vi "CRYSet ViewProperty Misc Front Panel.vi"(11 "Vi Ref":refnum<vi>) -> ()   [LabVIEW 2013]
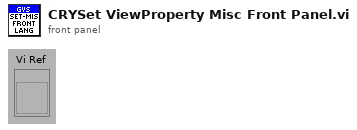
[diagram p1: front panel]
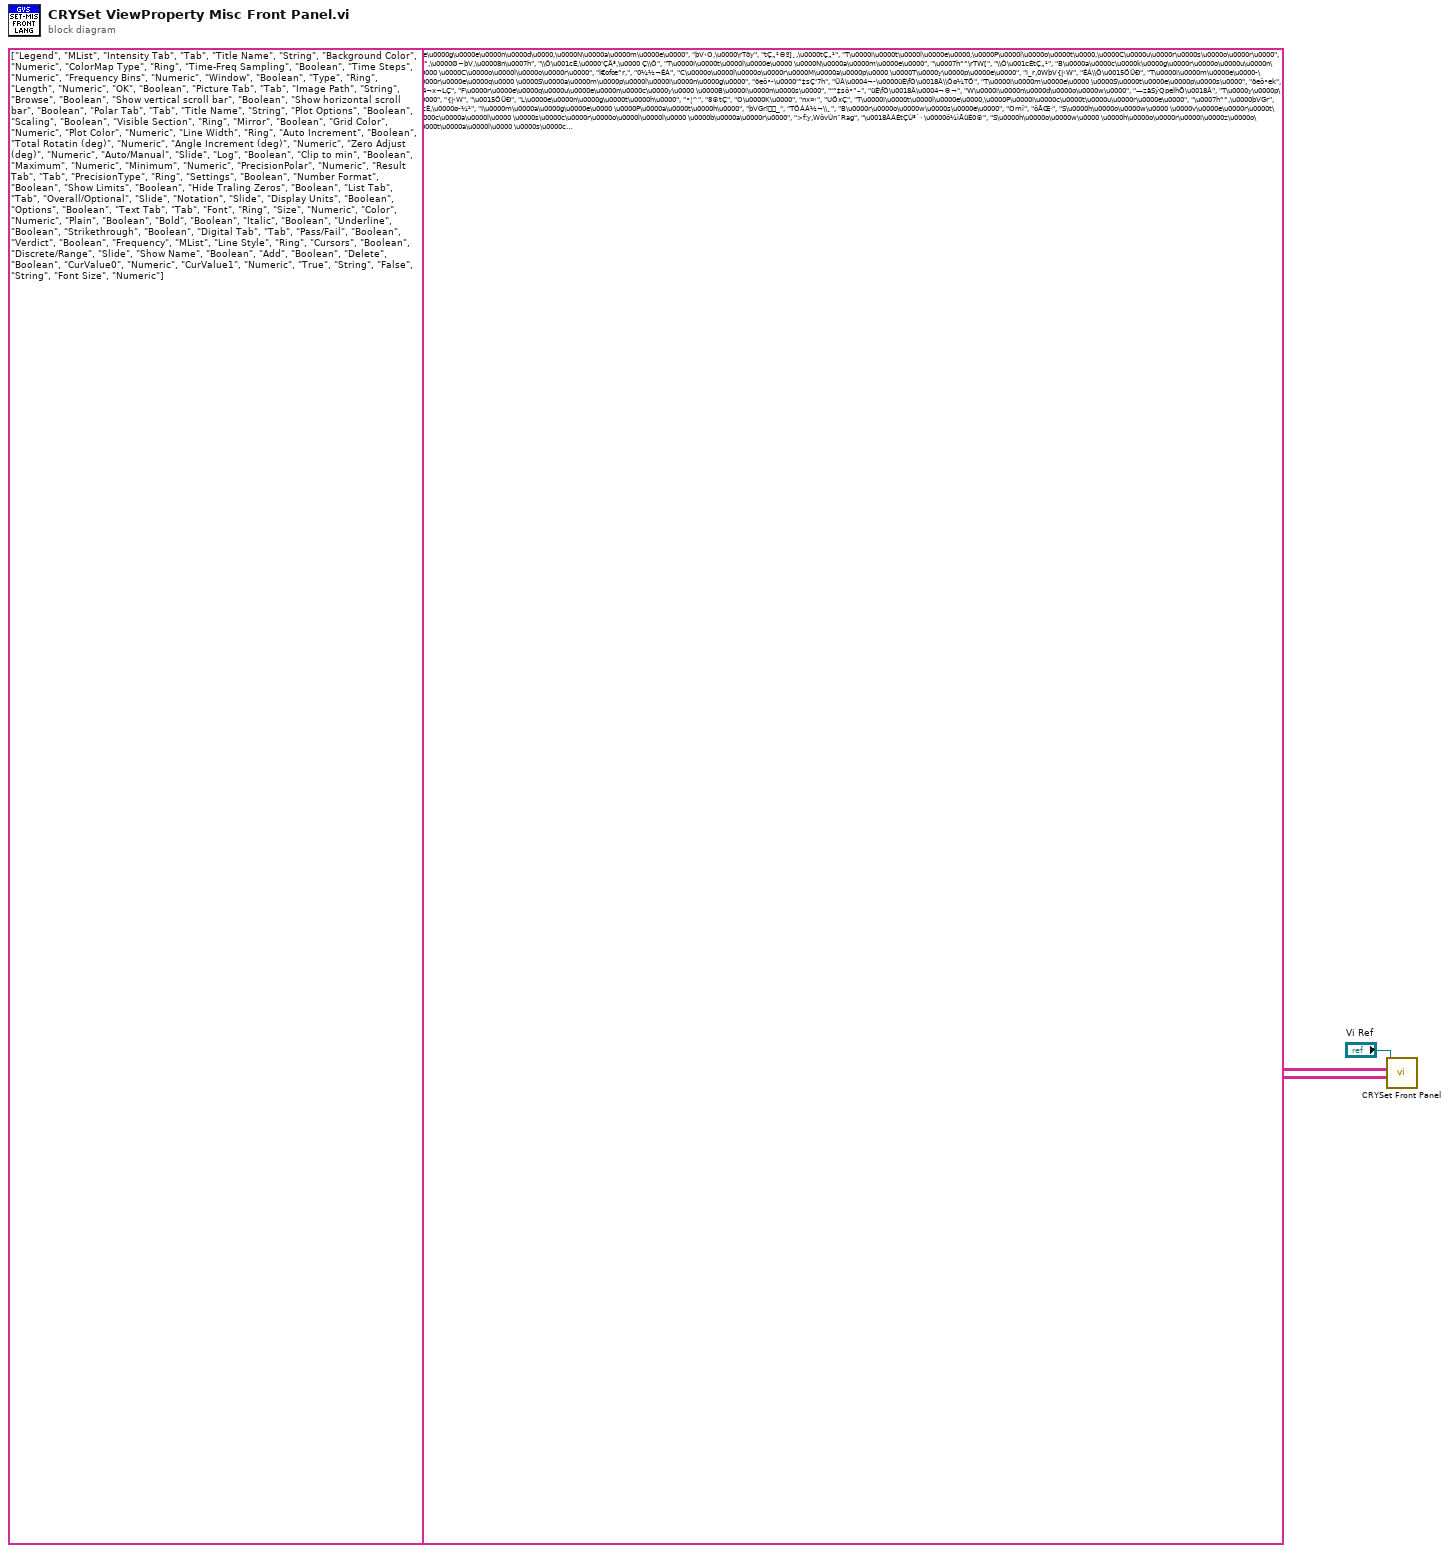
[diagram p0: block diagram]
diagram:
  # "Caption, Tab Page, Multilist Header, Button 4"
  # "Control Type"
  # "Control Name and Tab"
  # "caption, boolean text(,,,)"
  # "Caption/Boolean Text"
  n1 = call "CRYSet Front Panel.vi"("Caption(Boolean Text)"=string[][] [["L\u0000e\u0000g\u0000e\u0000n\u0000d\u0000,\u0000N\u0000a\u0000m\u0000e\u0000", "þV‹O,\u0000\rTðy", "tÇ„¹©º]¸,\u0000tÇ„¹"], ["T\u0000i\u0000t\u0000l\u0000e\u0000,\u0000P\u0000l\u0000o\u0000t\u0000,\u0000C\u0000u\u0000r\u0000s\u0000o\u0000r\u0000", "\u0007h˜˜,\u0000Ø~þV,\u00008n\u0007h", "\\Ô\u001cÈ,\u0000‘ÇÄ³,\u0000 Ç\\Ô"], ["T\u0000i\u0000t\u0000l\u0000e\u0000 \u0000N\u0000a\u0000m\u0000e\u0000", "\u0007h˜˜\rTW[", "\\Ô\u001cÈtÇ„¹"], ["B\u0000a\u0000c\u0000k\u0000g\u0000r\u0000o\u0000u\u0000n\u0000d\u0000 \u0000C\u0000o\u0000l\u0000o\u0000r\u0000", "Ì€ofœ˜r‚", "0¼½¬ÉÀ"], ["C\u0000o\u0000l\u0000o\u0000r\u0000M\u0000a\u0000p\u0000 \u0000T\u0000y\u0000p\u0000e\u0000", "i_r‚0WþV{|‹W", "ÉÀ\\Ô\u0015ÖÜÐ"], ["T\u0000i\u0000m\u0000e\u0000-\u0000F\u0000r\u0000e\u0000q\u0000 \u0000S\u0000a\u0000m\u0000p\u0000l\u0000i\u0000n\u0000g\u0000", "öeô•-\u0000‘˜‡sÇ‘7h", "ÜÂ\u0004¬-\u0000üÈ\fÓ\u0018Â\\Ôø¼TÖ"], ["T\u0000i\u0000m\u0000e\u0000 \u0000S\u0000t\u0000e\u0000p\u0000s\u0000", "öeô•ek", "ÜÂ\u0004¬x¬LÇ"], ["F\u0000r\u0000e\u0000q\u0000u\u0000e\u0000n\u0000c\u0000y\u0000 \u0000B\u0000i\u0000n\u0000s\u0000", "‘˜‡sô•”–", "üÈ\fÓ\u0018Â\u0004¬©¬"], ["W\u0000i\u0000n\u0000d\u0000o\u0000w\u0000", "—zãSýQpe", "=ÌhÕ\u0018Â"], ["T\u0000y\u0000p\u0000e\u0000", "{|‹W", "\u0015ÖÜÐ"], ["L\u0000e\u0000n\u0000g\u0000t\u0000h\u0000", "•¦^", "8®tÇ"], ["O\u0000K\u0000", "nx¤‹", "UÖxÇ"], ["T\u0000i\u0000t\u0000l\u0000e\u0000,\u0000P\u0000i\u0000c\u0000t\u0000u\u0000r\u0000e\u0000", "\u0007h˜˜,\u0000þVGr", "\\Ô\u001cÈ,\u0000ø­¼¹"], ["I\u0000m\u0000a\u0000g\u0000e\u0000 \u0000P\u0000a\u0000t\u0000h\u0000", "þVGrï_", "TÖÁÀ½¬\\¸"], ["B\u0000r\u0000o\u0000w\u0000s\u0000e\u0000", "Omȉ", "ôÅŒ·"], ["S\u0000h\u0000o\u0000w\u0000 \u0000v\u0000e\u0000r\u0000t\u0000i\u0000c\u0000a\u0000l\u0000 \u0000s\u0000c\u0000r\u0000o\u0000l\u0000l\u0000 \u0000b\u0000a\u0000r\u0000", ">f:y‚WôvÚn¨Rag", "\u0018ÂÁÉtÇÙ³`· \u0000ô¼ìÅüÈ0®"], ["S\u0000h\u0000o\u0000w\u0000 \u0000h\u0000o\u0000r\u0000i\u0000z\u0000o\u0000n\u0000t\u0000a\u0000l\u0000 \u0000s\u0000c\u0000r\u0000o\u0000l\u0000l\u0000 \u0000b\u0000a\u0000r\u0000", ">f:y4ls^Ún¨Rag", "\u0018ÂÉÓtÇÙ³`· \u0000ô¼ìÅüÈ0®"], ["T\u0000i\u0000t\u0000l\u0000e\u0000,\u0000P\u0000l\u0000o\u0000t\u0000,\u0000X\u0000Y\u0000 \u0000G\u0000r\u0000a\u0000p\u0000h\u0000", "\u0007h˜˜,\u0000Ø~þV,\u0000X\u0000Y\u0000þVhˆ", "\\Ô\u001cÈ,\u0000‘ÇÄ³,\u0000X\u0000Y\u0000ø­|·\u0004Õ"], ["T\u0000i\u0000t\u0000l\u0000e\u0000 \u0000N\u0000a\u0000m\u0000e\u0000", "\u0007h˜˜\rTW[", "\\Ô\u001cÈtÇ„¹"], ["P\u0000l\u0000o\u0000t\u0000 \u0000O\u0000p\u0000t\u0000i\u0000o\u0000n\u0000s\u0000", "Ø~þV\ty", "‘ÇÄ³ ÁÝÐmÕ©º"], ["S\u0000c\u0000a\u0000l\u0000i\u0000n\u0000g\u0000", ")>e", "™ÌÄ³"], ["V\u0000i\u0000s\u0000i\u0000b\u0000l\u0000e\u0000 \u0000S\u0000e\u0000c\u0000t\u0000i\u0000o\u0000n\u0000", "ïSÁè\u0006R", "ô¼„Çl­íÅ"], ["M\u0000i\u0000r\u0000r\u0000o\u0000r\u0000", "\\•P[ÍS\u0004\\", "p¬¸Æ\u0018¼¬À"], ["G\u0000r\u0000i\u0000d\u0000 \u0000C\u0000o\u0000l\u0000o\u0000r\u0000", "Q<hœ˜r‚", "©¬ÇÉÀ\b¬"], ["P\u0000l\u0000o\u0000t\u0000 \u0000C\u0000o\u0000l\u0000o\u0000r\u0000", "Ø~þVœ˜r‚", " Á \u0000ÉÀ\b¬"], ["L\u0000i\u0000n\u0000e\u0000 \u0000W\u0000i\u0000d\u0000t\u0000h\u0000", "Ø~þV¿~½[¦^", " Á \u0000\b±D¾"], ["A\u0000u\u0000t\u0000o\u0000 \u0000I\u0000n\u0000c\u0000r\u0000e\u0000m\u0000e\u0000n\u0000t\u0000", "ê¨RXÏ", "ÇÙ³É\u0000¬"], ["T\u0000o\u0000t\u0000a\u0000l\u0000 \u0000R\u0000o\u0000t\u0000a\u0000t\u0000i\u0000n\u0000 \u0000(\u0000d\u0000e\u0000g\u0000)\u0000", "hQSOÞVl(\u0000¦^)\u0000", "\u0004È´ÌŒÖ\u0004È(\u0000Ä³)\u0000"], ["A\u0000n\u0000g\u0000l\u0000e\u0000 \u0000I\u0000n\u0000c\u0000r\u0000e\u0000m\u0000e\u0000n\u0000t\u0000 \u0000(\u0000d\u0000e\u0000g\u0000)\u0000", "Ò‰¦^žXÏ‘(\u0000¦^)\u0000", "\u0001¬É½(\u0000Ä³)\u0000"], ["Z\u0000e\u0000r\u0000o\u0000 \u0000A\u0000d\u0000j\u0000u\u0000s\u0000t\u0000 \u0000(\u0000d\u0000e\u0000g\u0000)\u0000", "\u0003Œö–(\u0000¦^)\u0000", "9¸pÈ\bÈ(\u0000Ä³)\u0000"], ["A\u0000u\u0000t\u0000o\u0000/\u0000M\u0000a\u0000n\u0000u\u0000a\u0000l\u0000,\u0000A\u0000u\u0000t\u0000o\u0000,\u0000M\u0000a\u0000n\u0000u\u0000a\u0000l\u0000", "A\u0000u\u0000t\u0000o\u0000/\u0000M\u0000a\u0000n\u0000u\u0000a\u0000l\u0000,\u0000ê¨R,\u0000Kb¨R", "ÇÙ³/\u0000\u0018ÂÙ³,\u0000ÇÙ³,\u0000\u0018ÂÙ³"], ["L\u0000o\u0000g\u0000", "ù[pe", "\\¸ø­"], ["C\u0000l\u0000i\u0000p\u0000 \u0000t\u0000o\u0000 \u0000m\u0000i\u0000n\u0000", "jR\u0000gNO", "\\ÍÁÇ¹"], ["M\u0000a\u0000x\u0000i\u0000m\u0000u\u0000m\u0000", "\u0000g'Y<P", "\\Í\u0000³\u0012¬"], ["M\u0000i\u0000n\u0000i\u0000m\u0000u\u0000m\u0000", "\u0000g\u000f\\<P", "\\ÍŒÁ\u0012¬"], ["P\u0000r\u0000e\u0000c\u0000i\u0000s\u0000i\u0000o\u0000n\u0000", "¾|¦^", "\u0015È\u0000¼Ä³"], ["T\u0000i\u0000t\u0000l\u0000e\u0000,\u0000F\u0000o\u0000r\u0000m\u0000a\u0000t\u0000", "\u0007h˜˜,\u0000<h\u000f_", "\\Ô\u001cÈ,\u0000\u0015ÖÝÂ"], ["P\u0000r\u0000e\u0000c\u0000i\u0000s\u0000i\u0000o\u0000n\u0000T\u0000y\u0000p\u0000e\u0000,\u0000D\u0000i\u0000g\u0000i\u0000t\u0000a\u0000l\u0000s\u0000 \u0000o\u0000f\u0000 \u0000p\u0000r\u0000e\u0000c\u0000i\u0000s\u0000i\u0000o\u0000n\u0000,\u0000S\u0000i\u0000g\u0000n\u0000i\u0000f\u0000i\u0000c\u0000a\u0000n\u0000t\u0000 \u0000d\u0000i\u0000g\u0000i\u0000t\u0000s\u0000 \u0000", "¾|¦^,\u0000¾|¦^MOpe,\u0000\tgHepeW[", "\u0015È\u0000¼Ä³,\u0000D\u0000i\u0000g\u0000i\u0000t\u0000a\u0000l\u0000s\u0000 \u0000o\u0000f\u0000 \u0000p\u0000r\u0000e\u0000c\u0000i\u0000s\u0000i\u0000o\u0000n\u0000,\u0000S\u0000i\u0000g\u0000n\u0000i\u0000f\u0000i\u0000c\u0000a\u0000n\u0000t\u0000 \u0000d\u0000i\u0000g\u0000i\u0000t\u0000s\u0000 \u0000"], ["S\u0000e\u0000t\u0000t\u0000i\u0000n\u0000g\u0000s\u0000", "緥n", "$Á\u0015È"], ["N\u0000u\u0000m\u0000b\u0000e\u0000r\u0000 \u0000F\u0000o\u0000r\u0000m\u0000a\u0000t\u0000", "peW[<h\u000f_", "\u0018Â\u0012¬\u0015ÖÝÂ"], ["S\u0000h\u0000o\u0000w\u0000 \u0000L\u0000i\u0000m\u0000i\u0000t\u0000s\u0000", ">f:yP–6R", "\\ÕÄ¬ô¼ìÅüÈ0®"], ["H\u0000i\u0000d\u0000e\u0000 \u0000T\u0000r\u0000a\u0000i\u0000l\u0000i\u0000n\u0000g\u0000 \u0000Z\u0000e\u0000r\u0000o\u0000s\u0000", "Ï>\\ö", "9¸,¯¬¹(Â0®0®"], ["T\u0000i\u0000t\u0000l\u0000e\u0000,\u0000F\u0000o\u0000n\u0000t\u0000", "\u0007h˜˜,\u0000<h\u000f_", "\\Ô\u001cÈ,\u0000\u0015ÖÝÂ"], ["O\u0000v\u0000e\u0000r\u0000a\u0000l\u0000l\u0000/\u0000O\u0000p\u0000t\u0000i\u0000o\u0000n\u0000a\u0000l\u0000,\u0000O\u0000v\u0000e\u0000r\u0000a\u0000l\u0000l\u0000,\u0000O\u0000p\u0000t\u0000i\u0000o\u0000n\u0000a\u0000l\u0000", "O\u0000v\u0000e\u0000r\u0000a\u0000l\u0000l\u0000/\u0000O\u0000p\u0000t\u0000i\u0000o\u0000n\u0000a\u0000l\u0000,\u0000@b\tgÓ~g,\u0000\t[Ó~g", "O\u0000v\u0000e\u0000r\u0000a\u0000l\u0000l\u0000/\u0000O\u0000p\u0000t\u0000i\u0000o\u0000n\u0000a\u0000l\u0000,\u0000\u0004È´Ì,\u0000 ÁÝÐ"], ["N\u0000o\u0000t\u0000a\u0000t\u0000i\u0000o\u0000n\u0000,\u0000S\u0000I\u0000 \u0000N\u0000o\u0000t\u0000a\u0000t\u0000i\u0000o\u0000n\u0000,\u0000F\u0000l\u0000o\u0000a\u0000t\u0000i\u0000n\u0000g\u0000 \u0000p\u0000o\u0000i\u0000n\u0000t\u0000", "&{÷S,\u0000S\u0000I\u0000&{÷S,\u0000nm¹p", "\u0015ÖÝÂ,\u0000S\u0000I\u0000 \u0000\u0015ÖÝÂ,\u0000X¹\u0010È\u0018Â"], ["D\u0000i\u0000s\u0000p\u0000l\u0000a\u0000y\u0000 \u0000U\u0000n\u0000i\u0000t\u0000s\u0000", ">f:yUSMO", "è²\u0004Ç\u0004ÖÜÂ"], ["T\u0000a\u0000b\u0000l\u0000e\u0000 \u0000O\u0000p\u0000t\u0000i\u0000o\u0000n\u0000s\u0000", "h\ty", "\\Ô ÁÝÐmÕ©º"], ["T\u0000i\u0000t\u0000l\u0000e\u0000,\u0000F\u0000o\u0000r\u0000m\u0000a\u0000t\u0000", "\u0007h˜˜,\u0000W[SO", "\\Ô\u001cÈ,\u0000\u001cÁ´Ì"], ["F\u0000o\u0000n\u0000t\u0000", "W[SO", "\u001cÁ´Ì"], ["S\u0000i\u0000z\u0000e\u0000", ":\\ø[", "lÐ0®"], ["C\u0000o\u0000l\u0000o\u0000r\u0000", "œ˜r‚", "衫"], ["P\u0000l\u0000a\u0000i\u0000n\u0000", "¯~‡e,g", "ÉÓ8»"], ["B\u0000o\u0000l\u0000d\u0000", "—|SO", "\u0015¬pÈ"], ["I\u0000t\u0000a\u0000l\u0000i\u0000c\u0000", "œeSO", "¬À Á"], ["U\u0000n\u0000d\u0000e\u0000r\u0000l\u0000i\u0000n\u0000e\u0000", "\u000bN\u0012R¿~", "\u0011¼ Á"], ["S\u0000t\u0000r\u0000i\u0000k\u0000e\u0000t\u0000h\u0000r\u0000o\u0000u\u0000g\u0000h\u0000", " Rd–¿~", "\u0011É\u0004¬ Á"], ["T\u0000i\u0000t\u0000l\u0000e\u0000,\u0000P\u0000l\u0000o\u0000t\u0000", "\u0007h˜˜,\u0000Ø~þV", "\\Ô\u001cÈ,\u0000‘ÇÄ³"], ["P\u0000a\u0000s\u0000s\u0000/\u0000F\u0000a\u0000i\u0000l\u0000", "\u001aÇ/\u00001Y%", "\u0004ÈTÖtºô¼0®"], ["V\u0000e\u0000r\u0000d\u0000i\u0000c\u0000t\u0000,\u0000P\u0000a\u0000s\u0000s\u0000e\u0000d\u0000,\u0000F\u0000a\u0000i\u0000l\u0000e\u0000d\u0000", "V\u0000e\u0000r\u0000d\u0000i\u0000c\u0000t\u0000,\u0000\u001aÇ,\u00001Y%", "V\u0000e\u0000r\u0000d\u0000i\u0000c\u0000t\u0000,\u0000µÑü¬,\u0000äÂ(Ó"], ["F\u0000r\u0000e\u0000q\u0000u\u0000e\u0000n\u0000c\u0000y\u0000,\u0000F\u0000r\u0000e\u0000q\u0000u\u0000e\u0000n\u0000c\u0000y\u0000", "‘˜‡s,\u0000‘˜‡s", "üÈ\fÓ\u0018Â©º]¸,\u0000üÈ\fÓ\u0018Â"], ["L\u0000i\u0000n\u0000e\u0000 \u0000S\u0000t\u0000y\u0000l\u0000e\u0000,\u0000s\u0000o\u0000l\u0000i\u0000d\u0000,\u0000d\u0000a\u0000s\u0000h\u0000,\u0000d\u0000o\u0000t\u0000,\u0000d\u0000a\u0000s\u0000h\u0000d\u0000o\u0000t\u0000,\u0000d\u0000a\u0000s\u0000h\u0000d\u0000o\u0000t\u0000d\u0000o\u0000t\u0000", "¿~ag7h\u000f_,\u0000ž[¿~,\u0000Z†¿~,\u0000¹p¿~,\u0000¹p\u0012R¿~,\u0000ÌS¹p\u0012R¿~", " Á \u0000\u0015ÖÝÂ,\u0000s\u0000o\u0000l\u0000i\u0000d\u0000,\u0000d\u0000a\u0000s\u0000h\u0000,\u0000d\u0000o\u0000t\u0000,\u0000d\u0000a\u0000s\u0000h\u0000d\u0000o\u0000t\u0000,\u0000d\u0000a\u0000s\u0000h\u0000d\u0000o\u0000t\u0000d\u0000o\u0000t\u0000"], ["C\u0000u\u0000r\u0000s\u0000o\u0000r\u0000s\u0000", "8n\u0007h", " Ç\\Ô"], ["D\u0000i\u0000s\u0000c\u0000r\u0000e\u0000t\u0000e\u0000/\u0000R\u0000a\u0000n\u0000g\u0000e\u0000,\u0000D\u0000i\u0000s\u0000c\u0000r\u0000e\u0000t\u0000e\u0000,\u0000R\u0000a\u0000n\u0000g\u0000e\u0000", "»yce/\u0000\u0003ƒôV,\u0000»yce,\u0000\u0003ƒôV", "¬¹°À/\u0000”¼\u0004Ç,\u0000¬¹°À,\u0000”¼\u0004Ç"], ["S\u0000h\u0000o\u0000w\u0000 \u0000N\u0000a\u0000m\u0000e\u0000", ">f:y\rTW[", "tÇ„¹ \u0000ô¼ìÅüÈ0®"], ["A\u0000d\u0000d\u0000", "ý R", "”Í\u0000¬"], ["D\u0000e\u0000l\u0000e\u0000t\u0000e\u0000", " Rd–", "­À\u001cÈ"], ["S\u0000t\u0000a\u0000r\u0000t\u0000 \u0000F\u0000r\u0000e\u0000q\u0000", "\u0000_ËY‘˜‡s", "ÜÂ‘ÇüÈ\fÓ\u0018Â"], ["E\u0000n\u0000d\u0000 \u0000F\u0000r\u0000e\u0000q\u0000", "+g>\\‘˜‡s", "]°üÈ\fÓ\u0018Â"], ["T\u0000r\u0000u\u0000e\u0000", "\u001fw", "8Ì"], ["F\u0000a\u0000l\u0000s\u0000e\u0000", "GP", "p¬ÓÉ"], ["F\u0000o\u0000n\u0000t\u0000 \u0000S\u0000i\u0000z\u0000e\u0000", "W[SO'Y\u000f\\", "ðÓ¸ÒlÐ0®"]], "Control ID and Type(Label Name, Type)"=string[][] [["Legend", "MList"], ["Intensity Tab", "Tab"], ["Title Name", "String"], ["Background Color", "Numeric"], ["ColorMap Type", "Ring"], ["Time-Freq Sampling", "Boolean"], ["Time Steps", "Numeric"], ["Frequency Bins", "Numeric"], ["Window", "Boolean"], ["Type", "Ring"], ["Length", "Numeric"], ["OK", "Boolean"], ["Picture Tab", "Tab"], ["Image Path", "String"], ["Browse", "Boolean"], ["Show vertical scroll bar", "Boolean"], ["Show horizontal scroll bar", "Boolean"], ["Polar Tab", "Tab"], ["Title Name", "String"], ["Plot Options", "Boolean"], ["Scaling", "Boolean"], ["Visible Section", "Ring"], ["Mirror", "Boolean"], ["Grid Color", "Numeric"], ["Plot Color", "Numeric"], ["Line Width", "Ring"], ["Auto Increment", "Boolean"], ["Total Rotatin (deg)", "Numeric"], ["Angle Increment (deg)", "Numeric"], ["Zero Adjust (deg)", "Numeric"], ["Auto/Manual", "Slide"], ["Log", "Boolean"], ["Clip to min", "Boolean"], ["Maximum", "Numeric"], ["Minimum", "Numeric"], ["PrecisionPolar", "Numeric"], ["Result Tab", "Tab"], ["PrecisionType", "Ring"], ["Settings", "Boolean"], ["Number Format", "Boolean"], ["Show Limits", "Boolean"], ["Hide Traling Zeros", "Boolean"], ["List Tab", "Tab"], ["Overall/Optional", "Slide"], ["Notation", "Slide"], ["Display Units", "Boolean"], ["Options", "Boolean"], ["Text Tab", "Tab"], ["Font", "Ring"], ["Size", "Numeric"], ["Color", "Numeric"], ["Plain", "Boolean"], ["Bold", "Boolean"], ["Italic", "Boolean"], ["Underline", "Boolean"], ["Strikethrough", "Boolean"], ["Digital Tab", "Tab"], ["Pass/Fail", "Boolean"], ["Verdict", "Boolean"], ["Frequency", "MList"], ["Line Style", "Ring"], ["Cursors", "Boolean"], ["Discrete/Range", "Slide"], ["Show Name", "Boolean"], ["Add", "Boolean"], ["Delete", "Boolean"], ["CurValue0", "Numeric"], ["CurValue1", "Numeric"], ["True", "String"], ["False", "String"], ["Font Size", "Numeric"]], "Vi Ref"="Vi Ref") -> ()  [unwired: 9 in]
